vi "create_logarithmic_array.vi"(1 "Logarithmic Array":T1={"Initial Value"=1, "Fineness Factor"=1, "Number of Values"=10, "Generate Logarithmic\nArray?"=TRUE}) -> (0 "Generated Log Array":dbl[](array[numeric])=[1.0, 2.718281828459045, 7.38905609893065, 20.085536923187668, 54.598150033144236, 148.4131591025766, 403.4287934927351, 1096.6331584284585, 2980.9579870417283, 8103.083927575384, 0.0, 0.0, 0.0, 0.0, 0.0, 0.0, 0.0, 0.0, 0.0, 0.0])   [LabVIEW 2013]
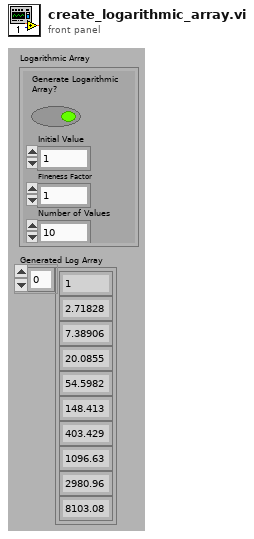
[diagram p1: front panel]
types:
  T1 = cluster{"Initial Value":i32, "Fineness Factor":i32, "Number of Values":i32, "Generate Logarithmic\nArray?":bool}
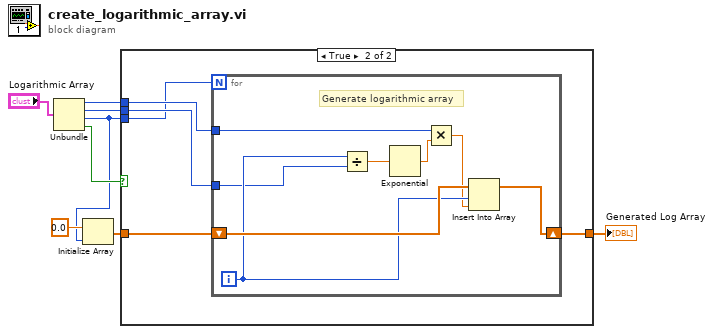
[diagram p0: block diagram]
diagram:
  n1 = Unbundle("Logarithmic Array") -> ("Initial Value"=w2:i32, "Fineness Factor"=w7:i32, "Number of Values"=w1:i32, "Generate Logarithmic\nArray?"=w6:bool)
  n2 = Initialize Array(0.0 ("element"), w1) -> (w4:dbl[])
  n3 = case shown="True" w6 {
    tunnel: w2 -> [_ w14]
    tunnel: w7 -> [_ w13]
    tunnel: w1 -> [_ w12]
    tunnel: [w9 w11] -> w5
    tunnel: w4 -> [w9 w10]
    frame False {
      # "Don't generate logarithmic array"
    }
    frame True {
      n4 = for {
        N: w12 -> [_]
        shift-right: [w19] -> w11
        shift-left: w10 -> [w21]
        tunnel: w14 -> [w17]
        tunnel: w13 -> [w15]
        i -> [w20]
        # "Generate logarithmic array"
        n5 = Divide(x=w20, y=w15) -> (x/y=w22:dbl)
        n6 = Exponential(1:w22) -> (0:w18:dbl)
        n7 = Multiply(x=w17, y=w18) -> (x*y=w16:dbl)
        n8 = Insert Into Array(array=w21, index=w20, new element=w16) -> (w19:dbl[])
      }
    }
  }
  "Generated Log Array" <- w5
